vi "Teleop - Serializer stop (SubVI).vi"(9 "Constant Cluster In":T1 {"32. shooterHoodAngleRange" format="%_6f"; "31. turretAngleRange" format="%_6f"; "30. shooterVelocityLowerLimit" format="%_6f"; "29. shooterVelocityUpperLimit" format="%_6f"; "28. Robot Track Width (inches)" format="%_6f"; "27. Shooter Spin Up Speed (RPM)" format="%_6f"; "26. Climb Down Speed %" format="%_6f"; "25. Climb Up Speed %" format="%_6f"; "24. Intake Continue Time (s)" format="%_6f"; "23. Intake Spit Speed %" format="%_6f"; "22. Intake Suck Speed %" format="%_6f"; "21. CP Wheel Diameter" format="%_6f"; "20. Clockwise CP Fudge" format="%_6f"; "19. CouterClockwise CP Fudge" format="%_6f"; "18. Inches per Sector" format="%_6f"; "17. Ticks/Rotation Neo 550" format="%_6f"; "16. Control Panel Wheel Diameter" format="%_6f"; "15. Center-Center Sector Distance" format="%_6f"; "14. Inches / Tick Drivetrain" format="%_6f"; "13. Auton I Output Limit Drive Straight Gain" format="%_6f"; "12. Auton Deriv Drive Straight Gain" format="%_6f"; "11. Auton Int Drive Straight Gain" format="%_6f"; "10. Auton Prop Drive Straight Gain" format="%_6f"; "9. Auton I Output Limit Turn Gain" format="%_6f"; "8. Auton Deriv Turn Gain" format="%_6f"; "7. Auton Int Turn Gain" format="%_6f"; "1. Auton Prop Drive Gain" format="%_6f"; "2. Auton Int Drive Gain" format="%_6f"; "3. Auton Deriv Drive Gain" format="%_6f"; "4. I Output Drive  Limit" format="%_6f"; "5. Auto Drive Cheat (%)" format="%_6f"; "6. Auton Prop Turn Gain" format="%_6f"}, 10 "serializerSpinVelocity in":dbl, 11 "was there a clicked button?":bool) -> (1 "Constant Cluster Out":T1 {"32. shooterHoodAngleRange" format="%_6f"; "31. turretAngleRange" format="%_6f"; "30. shooterVelocityLowerLimit" format="%_6f"; "29. shooterVelocityUpperLimit" format="%_6f"; "28. Robot Track Width (inches)" format="%_6f"; "27. Shooter Spin Up Speed (RPM)" format="%_6f"; "26. Climb Down Speed %" format="%_6f"; "25. Climb Up Speed %" format="%_6f"; "24. Intake Continue Time (s)" format="%_6f"; "23. Intake Spit Speed %" format="%_6f"; "22. Intake Suck Speed %" format="%_6f"; "21. CP Wheel Diameter" format="%_6f"; "20. Clockwise CP Fudge" format="%_6f"; "19. CouterClockwise CP Fudge" format="%_6f"; "18. Inches per Sector" format="%_6f"; "17. Ticks/Rotation Neo 550" format="%_6f"; "16. Control Panel Wheel Diameter" format="%_6f"; "15. Center-Center Sector Distance" format="%_6f"; "14. Inches / Tick Drivetrain" format="%_6f"; "13. Auton I Output Limit Drive Straight Gain" format="%_6f"; "12. Auton Deriv Drive Straight Gain" format="%_6f"; "11. Auton Int Drive Straight Gain" format="%_6f"; "10. Auton Prop Drive Straight Gain" format="%_6f"; "9. Auton I Output Limit Turn Gain" format="%_6f"; "8. Auton Deriv Turn Gain" format="%_6f"; "7. Auton Int Turn Gain" format="%_6f"; "1. Auton Prop Drive Gain" format="%_6f"; "2. Auton Int Drive Gain" format="%_6f"; "3. Auton Deriv Drive Gain" format="%_6f"; "4. I Output Drive  Limit" format="%_6f"; "5. Auto Drive Cheat (%)" format="%_6f"; "6. Auton Prop Turn Gain" format="%_6f"}, 2 "serializerSpinVelocity out":dbl)   [LabVIEW 2019]
uses:
  Disabled/Constant VI_s/Disabled - Constant Cluster Typedef.ctl
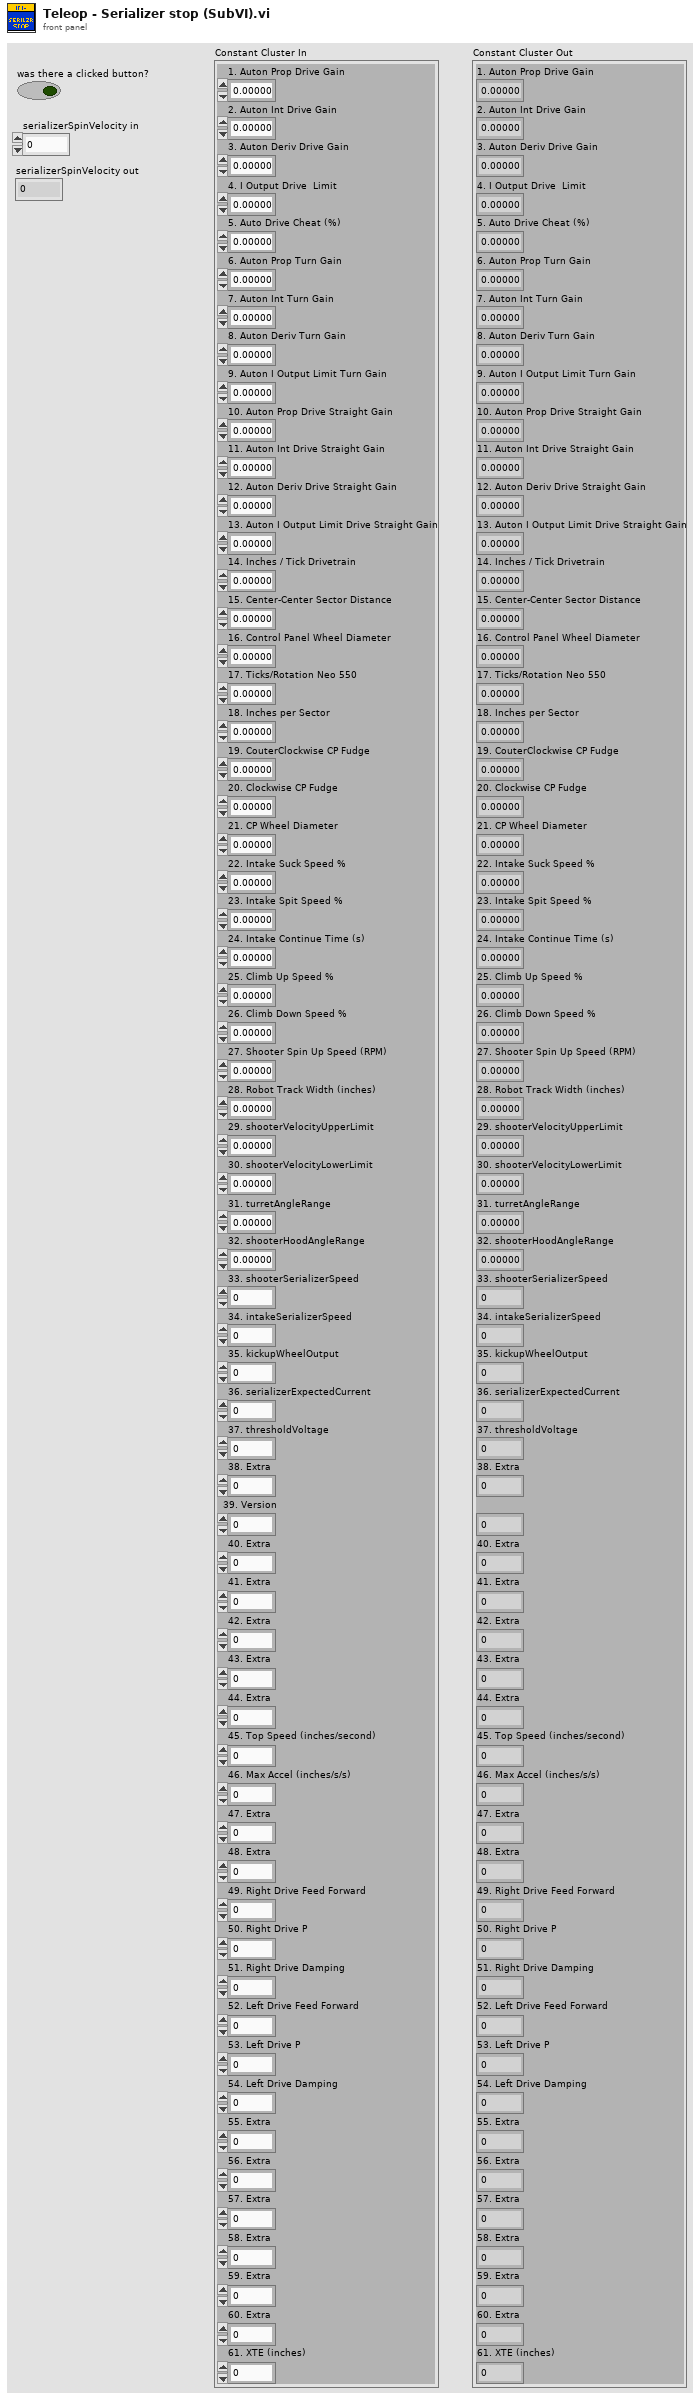
[diagram p1: front panel]
types:
  T1 = typedef "Disabled - Constant Cluster Typedef.ctl" = cluster{"1. Auton Prop Drive Gain":dbl, "2. Auton Int Drive Gain":dbl, "3. Auton Deriv Drive Gain":dbl, "4. I Output Drive  Limit":dbl, "5. Auto Drive Cheat (%)":dbl, "6. Auton Prop Turn Gain":dbl, "7. Auton Int Turn Gain":dbl, "8. Auton Deriv Turn Gain":dbl, "9. Auton I Output Limit Turn Gain":dbl, "10. Auton Prop Drive Straight Gain":dbl, "11. Auton Int Drive Straight Gain":dbl, "12. Auton Deriv Drive Straight Gain":dbl, "13. Auton I Output Limit Drive Straight Gain":dbl, "14. Inches / Tick Drivetrain":dbl, "15. Center-Center Sector Distance":dbl, "16. Control Panel Wheel Diameter":dbl, "17. Ticks/Rotation Neo 550":dbl, "18. Inches per Sector":dbl, "19. CouterClockwise CP Fudge":dbl, "20. Clockwise CP Fudge":dbl, "21. CP Wheel Diameter":dbl, "22. Intake Suck Speed %":dbl, "23. Intake Spit Speed %":dbl, "24. Intake Continue Time (s)":dbl, "25. Climb Up Speed %":dbl, "26. Climb Down Speed %":dbl, "27. Shooter Spin Up Speed (RPM)":dbl, "28. Robot Track Width (inches)":dbl, "29. shooterVelocityUpperLimit":dbl, "30. shooterVelocityLowerLimit":dbl, "31. turretAngleRange":dbl, "32. shooterHoodAngleRange":dbl, "33. shooterSerializerSpeed":dbl, "34. intakeSerializerSpeed":dbl, "35. kickupWheelOutput":dbl, "36. serializerExpectedCurrent":dbl, "37. thresholdVoltage":dbl, "38. Extra":dbl, "39. Version":dbl, "40. Extra":dbl, "41. Extra":dbl, "42. Extra":dbl, "43. Extra":dbl, "44. Extra":dbl, "45. Top Speed (inches/second)":dbl, "46. Max Accel (inches/s/s)":dbl, "47. Extra":dbl, "48. Extra":dbl, "49. Right Drive Feed Forward":dbl, "50. Right Drive P":dbl, "51. Right Drive Damping":dbl, "52. Left Drive Feed Forward":dbl, "53. Left Drive P":dbl, "54. Left Drive Damping":dbl, "55. Extra":dbl, "56. Extra":dbl, "57. Extra":dbl, "58. Extra":dbl, "59. Extra":dbl, "60. Extra":dbl, "61. XTE (inches)":dbl}
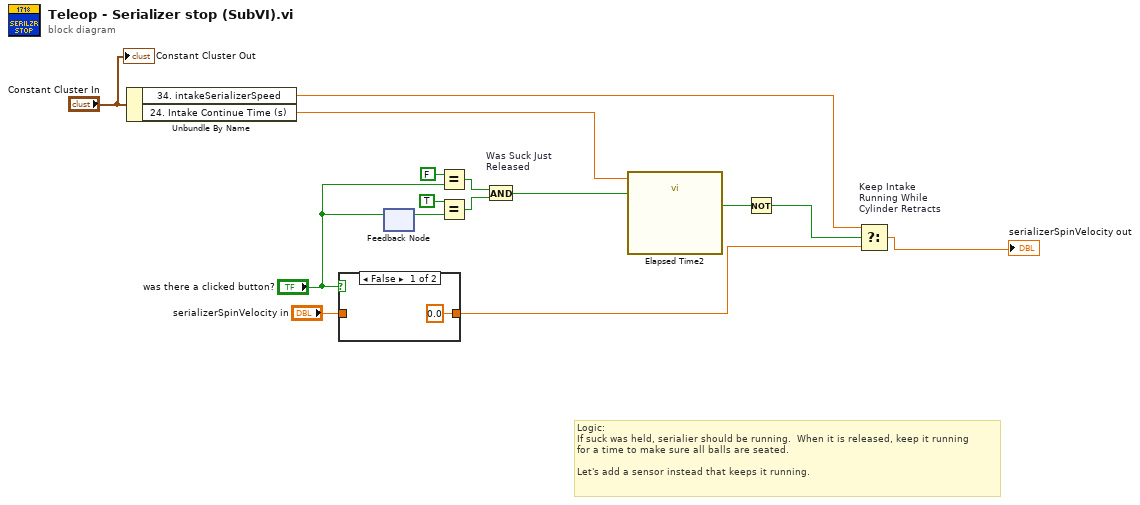
[diagram p0: block diagram]
diagram:
  # "Logic:\nIf suck was held, serialier should be running.  When it is released, keep it running\nfor a time to make sure all balls are seated.\n\nLet's add a sensor instead that keeps it running."
  n1 = Unbundle By Name("Constant Cluster In") -> ("34. intakeSerializerSpeed"=w2:dbl, "24. Intake Continue Time (s)"=w7:dbl)
  n2 = case shown="False" "was there a clicked button?" {
    tunnel: "serializerSpinVelocity in" -> [_ w17]
    tunnel: [0.0 ("serializerSpinVelocity") w17] -> w4
    frame False {
    }
    frame True {
    }
  }
  n3 = feedback #1() -> (w12:bool)  [unwired: 1 in]
  n4 = feedback-in #1("was there a clicked button?") -> ()
  n5 = Equal?(x=FALSE, y="was there a clicked button?") -> (x = y?=w10:bool)
  n6 = Equal?(x=TRUE, y=w12) -> (x = y?=w9:bool)
  n7 = And "Was Suck Just\nReleased"(x=w10, y=w9) -> (x .and. y?=w8:bool)
  n8 = call "Elapsed Time2"("Time Target (s)"=w7, "Reset"=w8) -> ("Time has Elapsed"=w6:bool)  [unwired: 10 in, 7 out]
  n9 = Not(x=w6) -> (.not. x?=w5:bool)
  n10 = Select "Keep Intake\nRunning While\nCylinder Retracts"(t=w2, s=w5, f=w4) -> (s? t:f=→"serializerSpinVelocity out":dbl)
  "Constant Cluster Out" <- "Constant Cluster In"
